vi "Configure serial port.vi"(8 "error in (no error)":errorcluster, 11 "Yudian AI - Serial Port Parameters":T1={"Baud rate"=enum."9600", "Parity"=enum."None", "Data bits"=8, "Flow Control"=enum."None", "Stop Bits"=enum."2", "Timeout (Sec)"=10, "termination char"=10, "Enable Termination"=FALSE, "VISA resource name"="COM4"} {"termination char" format="%.0x"; "Data bits" min=7 max=8 step=1}) -> (0 "error out":errorcluster, 3 "VISA resource name out":refnum<visa-resource-name>)   [LabVIEW 2010]
uses:
  <vilib>/Instr/_visa.llb/VISA Flush IO Buffer Mask.ctl
  <vilib>/Instr/_visa.llb/VISA Configure Serial Port (Instr).vi
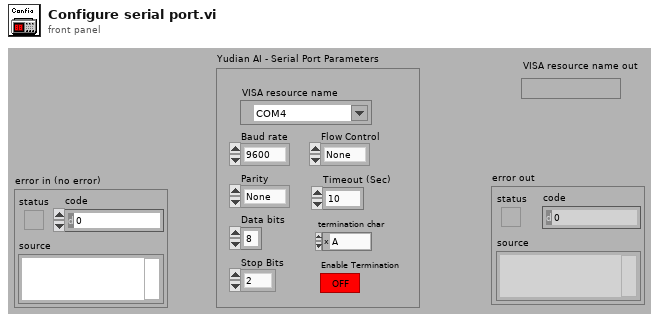
[diagram p1: front panel]
types:
  T1 = cluster{"Baud rate":enum16{"300", "600", "1200", "2400", "4800", "9600", "19200", "38400", "57600"}, "Parity":enum16{"None", "Odd", "Even", "Mark", "Space"}, "Data bits":u16, "Flow Control":enum16{"None", "X-OFF", "RTS / CTS"}, "Stop Bits":enum16{"1", "1.5", "2"}, "Timeout (Sec)":u32, "termination char":u8, "Enable Termination":bool, "VISA resource name":refnum<visa-resource-name>}
  T2 = typedef "VISA Flush IO Buffer Mask.ctl" = u16
  T3 = enum16{"300", "600", "1200", "2400", "4800", "9600", "19200", "38400", "57600"}
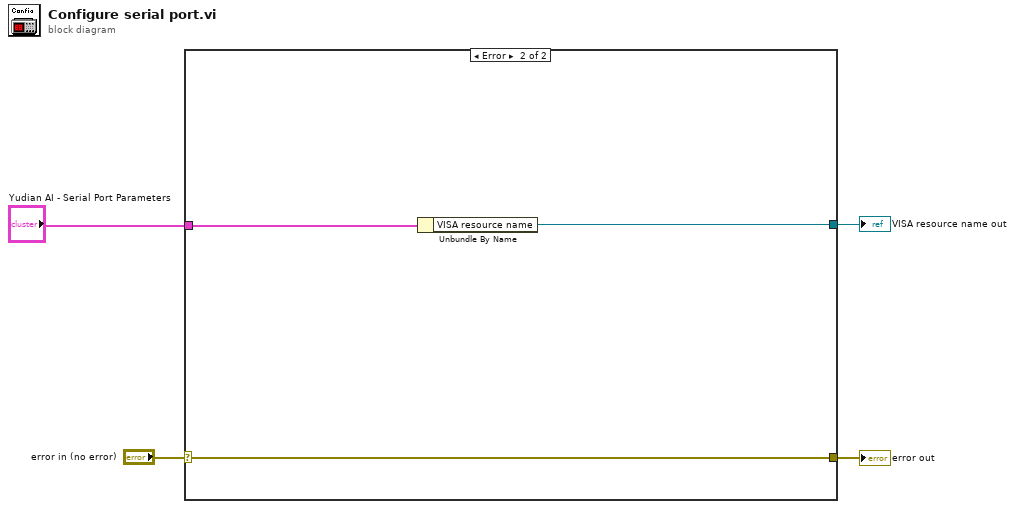
[diagram p0: block diagram]
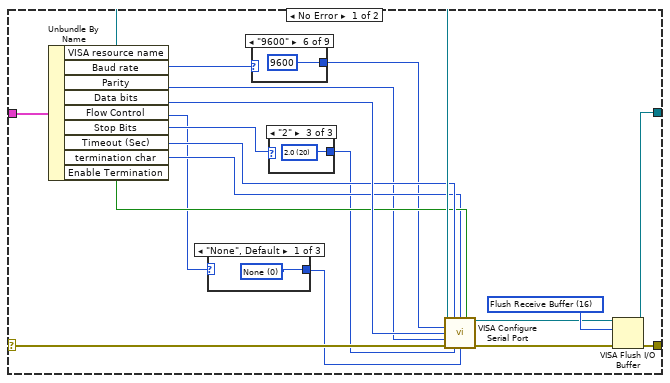
[diagram p2: hidden frame]
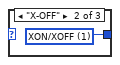
[diagram p3: hidden frame]
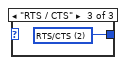
[diagram p4: hidden frame]
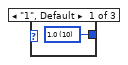
[diagram p5: hidden frame]
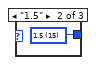
[diagram p6: hidden frame]
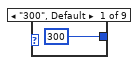
[diagram p7: hidden frame]
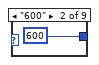
[diagram p8: hidden frame]
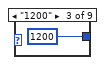
[diagram p9: hidden frame]
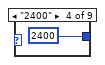
[diagram p10: hidden frame]
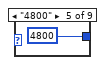
[diagram p11: hidden frame]
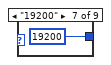
[diagram p12: hidden frame]
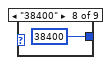
[diagram p13: hidden frame]
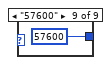
[diagram p14: hidden frame]
diagram:
  n1 = case shown="Error" "error in (no error)" {
    selector: "error in (no error)" -> [w14 w39]
    tunnel: [w7 w39] -> w3
    tunnel: "Yudian AI - Serial Port Parameters" -> [w22 w41]
    tunnel: [w5 w40] -> w2
    frame No Error {
      w9 = T2 16 items=["Flush Receive Buffer"=16, "Write Transmit Buffer to Device"=32, "Flush Receive Buffer (No I/O)"=64, "Flush Transmit Buffer"=128] ("Mask")
      n2 = Unbundle By Name(w22) -> ("VISA resource name"=w20:refnum<visa-resource-name>, "Baud rate"=w21:T3, "Parity"=w15:enum16{"None", "Odd", "Even", "Mark", "Space"}, "Data bits"=w19:u16, "Flow Control"=w11:enum16{"None", "X-OFF", "RTS / CTS"}, "Stop Bits"=w23:enum16{"1", "1.5", "2"}, "Timeout (Sec)"=w18:u32, "termination char"=w16:u8, "Enable Termination"=w17:bool)
      n3 = case shown="\"None\", Default" w11 {
        tunnel: [w24 w25 w26] -> w10
        frame "None", Default {
          w24 = u16 0 items=["None", "XON/XOFF", "RTS/CTS", "XON/XOFF & RTS/CTS", "DTR/DSR", "XON/XOFF & DTR/DSR"] ("flow control (0:none)")
        }
        frame "X-OFF" {
          w25 = u16 1 items=["None", "XON/XOFF", "RTS/CTS", "XON/XOFF & RTS/CTS", "DTR/DSR", "XON/XOFF & DTR/DSR"] ("flow control (0:none)")
        }
        frame "RTS / CTS" {
          w26 = u16 2 items=["None", "XON/XOFF", "RTS/CTS", "XON/XOFF & RTS/CTS", "DTR/DSR", "XON/XOFF & DTR/DSR"] ("flow control (0:none)")
        }
      }
      n4 = case shown="\"9600\"" w21 {
        tunnel: [u32 300 u32 600 u32 1200 u32 2400 u32 4800 u32 9600 u32 19200 u32 38400 u32 57600] -> w13
        frame "300", Default {
        }
        frame "600" {
        }
        frame "1200" {
        }
        frame "2400" {
        }
        frame "4800" {
        }
        frame "9600" {
        }
        frame "19200" {
        }
        frame "38400" {
        }
        frame "57600" {
        }
      }
      n5 = case shown="\"2\"" w23 {
        tunnel: [w27 w28 w29] -> w12
        frame "1", Default {
          w27 = u16 10 items=["1.0"=10, "1.5"=15, "2.0"=20] ("stop bits (10: 1 bit)")
        }
        frame "1.5" {
          w28 = u16 15 items=["1.0"=10, "1.5"=15, "2.0"=20] ("stop bits (10: 1 bit)")
        }
        frame "2" {
          w29 = u16 20 items=["1.0"=10, "1.5"=15, "2.0"=20] ("stop bits (10: 1 bit)")
        }
      }
      n6 = call-poly "VISA Configure Serial Port"("VISA resource name"=w20, "timeout (10sec)"=w18, "termination char\n(0xA = '\\n' = LF)"=w16, "Enable Termination\nChar (T)"=w17, "baud rate (9600)"=w13, "data bits (8)"=w19, "parity (0:none)"=w15, "error in (no error)"=w14, "stop bits (10: 1 bit)"=w12, "flow control (0:none)"=w10) -> ("VISA resource name out"=w6:refnum<visa-resource-name>, "error out"=w8:errorcluster)  [unwired: 4 in]
      n7 = VISA Flush I/O Buffer(VISA resource name=w6, mask (16)=w9, error in (no error)=w8) -> (VISA resource name out=w5:refnum<visa-resource-name>, error out=w7:errorcluster)
    }
    frame Error {
      n8 = Unbundle By Name(w41) -> ("VISA resource name"=w40:refnum<visa-resource-name>)
    }
  }
  "error out" <- w3
  "VISA resource name out" <- w2
